vi "OptimizeMaxVel.vi"(8 "error in (no error)":errorcluster, 11 "TapeDrive in":refnum<class "TapeDrive.lvclass">) -> (0 "error out":errorcluster, 1 "maxVel":dbl[](graph), 3 "TapeDrive out":refnum<class "TapeDrive.lvclass">)   [LabVIEW 2020, in "TapeDrive.lvclass"]
uses:
  TapeDrive.lvclass
  Ramp Pattern by Delta.vi
  NI_AALBase.lvlib
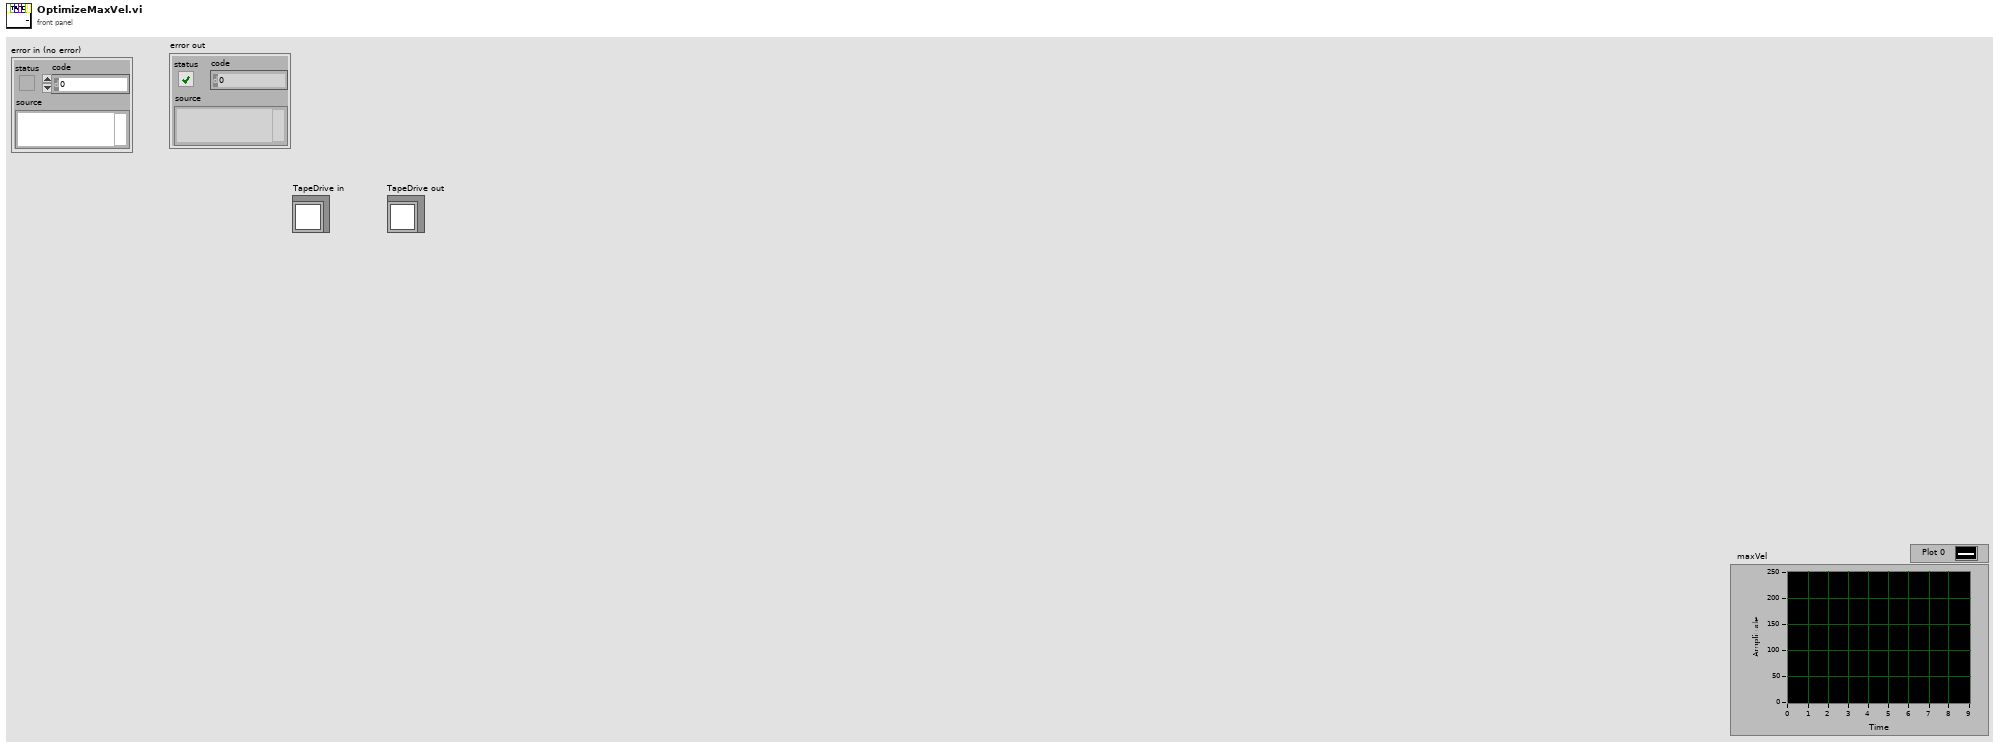
[diagram p1: front panel]
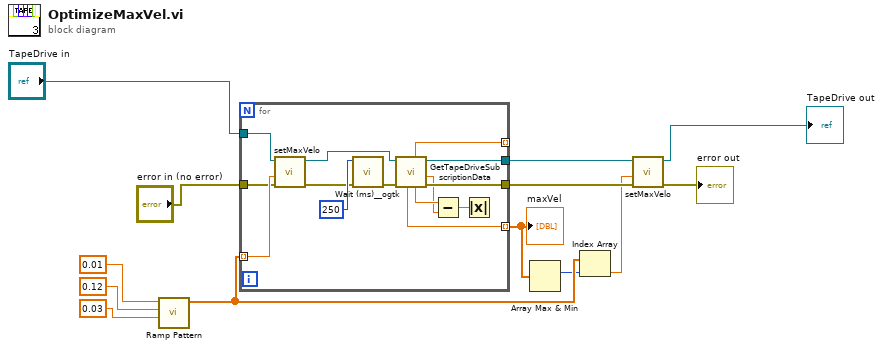
[diagram p0: block diagram]
diagram:
  n1 = call-poly "Ramp Pattern.vi"("start"=0.03, "end"=0.12, "delta"=0.01) -> ("Ramp Pattern"=w11:dbl[])  [unwired: 6 in, 2 out]
  n2 = for {
    tunnel: w11 -> [w27] mode=indexing
    tunnel: "TapeDrive in" -> [w16]
    tunnel: [w26] -> w3
    tunnel: [w25] -> _ mode=indexing
    tunnel: [w17] -> w10 mode=indexing
    tunnel: [w21] -> w13
    tunnel: "error in (no error)" -> [w15]
    n3 = call "setMaxVelo.vi"("error in (no error)"=w15, "NewVal"=w27, "TapeDrive in"=w16) -> ("error out"=w22:errorcluster, "TapeDrive out"=w14:refnum<class "TapeDrive.lvclass">)  [unwired: 6 in, 1 out]
    n4 = call "Wait (ms)__ogtk.vi"("error in (no error)"=w22, "milliseconds to wait"=u32 250) -> ("error out"=w24:errorcluster)  [unwired: 8 in, 1 out]
    n5 = call "GetTapeDriveSubscriptionData.vi"("error in (no error)"=w24, "TapeDrive in"=w14) -> ("error out"=w21:errorcluster, "TapeMonTargetY"=w19:dbl, "TapeDrive in 2"=w26:refnum<class "TapeDrive.lvclass">, "TapeMonCentroidY"=w20:dbl, "TapeMonCentroidX"=w25:dbl, "TapeMonMaxCounts"=w17:dbl)  [unwired: 3 in, 1 out]
    n6 = Subtract(x=w20, y=w19) -> (x-y=w18:dbl)
    n7 = Absolute Value(x=w18) -> ()  [unwired: 1 out]
  }
  "maxVel" <- w10
  n8 = Array Max & Min(array=w10) -> (max index (indices)=w6:i32)  [unwired: 3 out]
  n9 = Index Array(array=w11, index=w6) -> (element=w12:dbl)
  n10 = call "setMaxVelo.vi"("error in (no error)"=w13, "NewVal"=w12, "TapeDrive in"=w3) -> ("error out"=→"error out":errorcluster, "TapeDrive out"=→"TapeDrive out":refnum<class "TapeDrive.lvclass">)  [unwired: 6 in, 1 out]
